vi "svx_Polar_To_XY.vi"(11 "polar plot":T1) -> (0 "attribute out":variant, 1 "time/rev/RPM":dbl[](array[numeric]), 2 "y":dbl[](array[numeric]), 3 "x":dbl[](array[numeric]))   [LabVIEW 2017, in "SVX Polar Plot.xctl"]
uses:
  <vilib>/addons/_XControls/Polar Plot/SVX Polar Plot.xctl
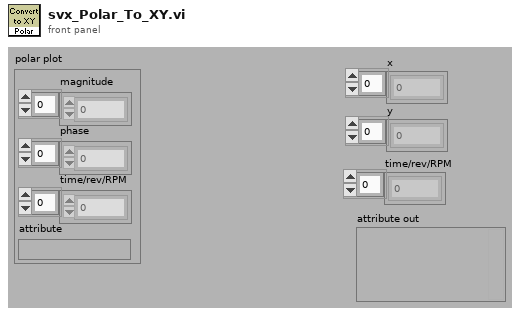
[diagram p1: front panel]
types:
  T1 = cluster{"magnitude":dbl[], "phase":dbl[], "time/rev/RPM":dbl[], "attribute":variant}
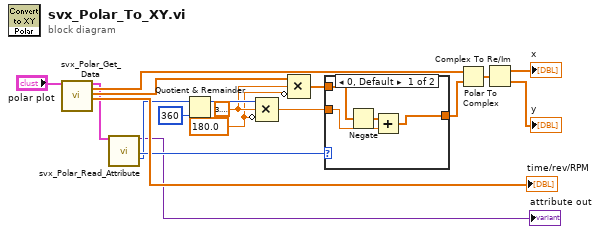
[diagram p0: block diagram]
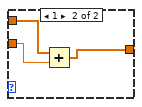
[diagram p2: hidden frame]
diagram:
  w11 = 180.0 ("value")
  w12 = 3.141592653589793
  n1 = call <vilib>:"svx_Polar_Get_Data.vi"("polar plot"="polar plot") -> ("polar plot out"=w5:T1, "magnitude"=w6:dbl[], "phase"=w7:dbl[], "time/rev/RPM"=→"time/rev/RPM":dbl[])  [unwired: 13 in, 2 out]
  n2 = call <vilib>:"svx_Polar_Read_Attribute.vi"("polar plot"=w5) -> ("attribute out"=→"attribute out":variant, "shaft rotating direction"=w4:u16, "probe angle [deg]"=w3:u16)  [unwired: 13 in, 3 out]
  n3 = Quotient & Remainder(x=w3, y=u16 360) -> (x-y*floor(x/y)=w17:u16)  [unwired: 1 out]
  n4 = Compound Arithmetic op=MULTIPLY(w17, w12, invert w11) -> (w15:dbl)
  n5 = Compound Arithmetic op=MULTIPLY(w7, w12, invert w11) -> (w13:dbl[])
  n6 = case shown="0, Default" w4 {
    tunnel: w15 -> [w22 w25]
    tunnel: w13 -> [w21 w24]
    tunnel: [w19 w23] -> w14
    frame 0, Default {
      n7 = Negate(x=w21) -> (-x=w20:dbl[])
      n8 = Add(x=w20, y=w22) -> (x+y=w19:dbl[])
    }
    frame 1 {
      n9 = Add(x=w24, y=w25) -> (x+y=w23:dbl[])
    }
  }
  n10 = Polar To Complex(1:w14, 2:w6) -> (0:w18:cdb[])
  n11 = Complex To Re/Im(x + iy=w18) -> (x=→"x":dbl[], y=→"y":dbl[])
